vi "Draw Line - Octant 1.vi"(5 "Delta y":i32, 6 "Colour":u32(colorbox), 7 "Delta x":i32, 8 "x Direction":i32, 9 "Y0":i32, 10 "X0":i32, 11 "Pixel Data in":u32[][](array[numeric])) -> (3 "Pixel Data out":u32[][](array[numeric]))   [LabVIEW 2022 SP3, in "Raster.lvlib"]
uses:
  Raster.lvlib
  Utility/Convert Pixels To Picture.vi/d601d993-a776-4dc8-89c7-357d8398c88c.vi
  Utility/Convert Pixels To Picture.vi/7816d0d6-8e4d-41a2-85ac-ed82f1435763.vi
  <vilib>/Utility/High Resolution Relative Seconds.vi
  <vilib>/picture/picture.llb/Draw Unflattened Pixmap.vi
  <vilib>/picture/picture.llb/Draw True-Color Pixmap.vi
  Utility/Utility.lvlib
panel:
  out "new picture 2":picture
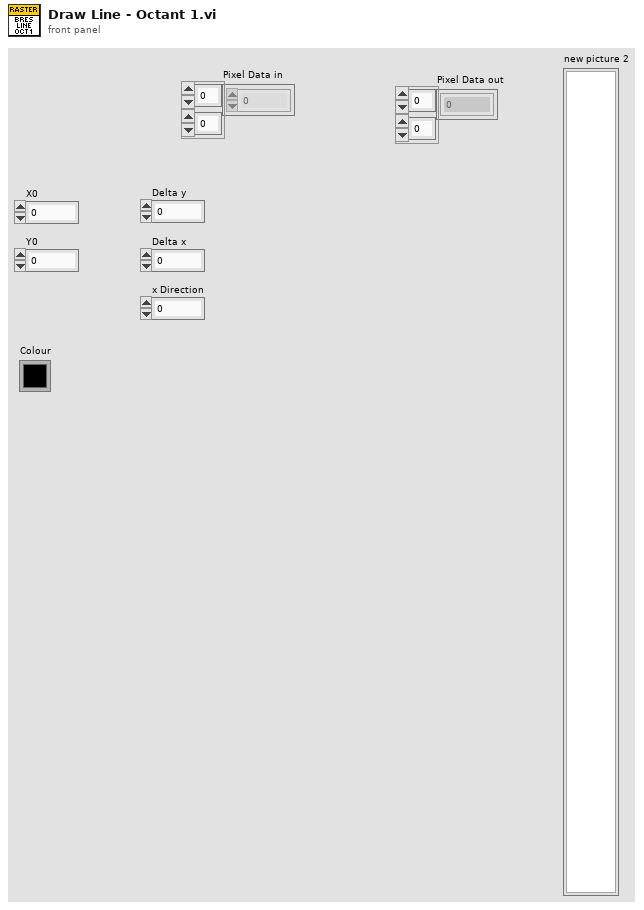
[diagram p1: front panel]
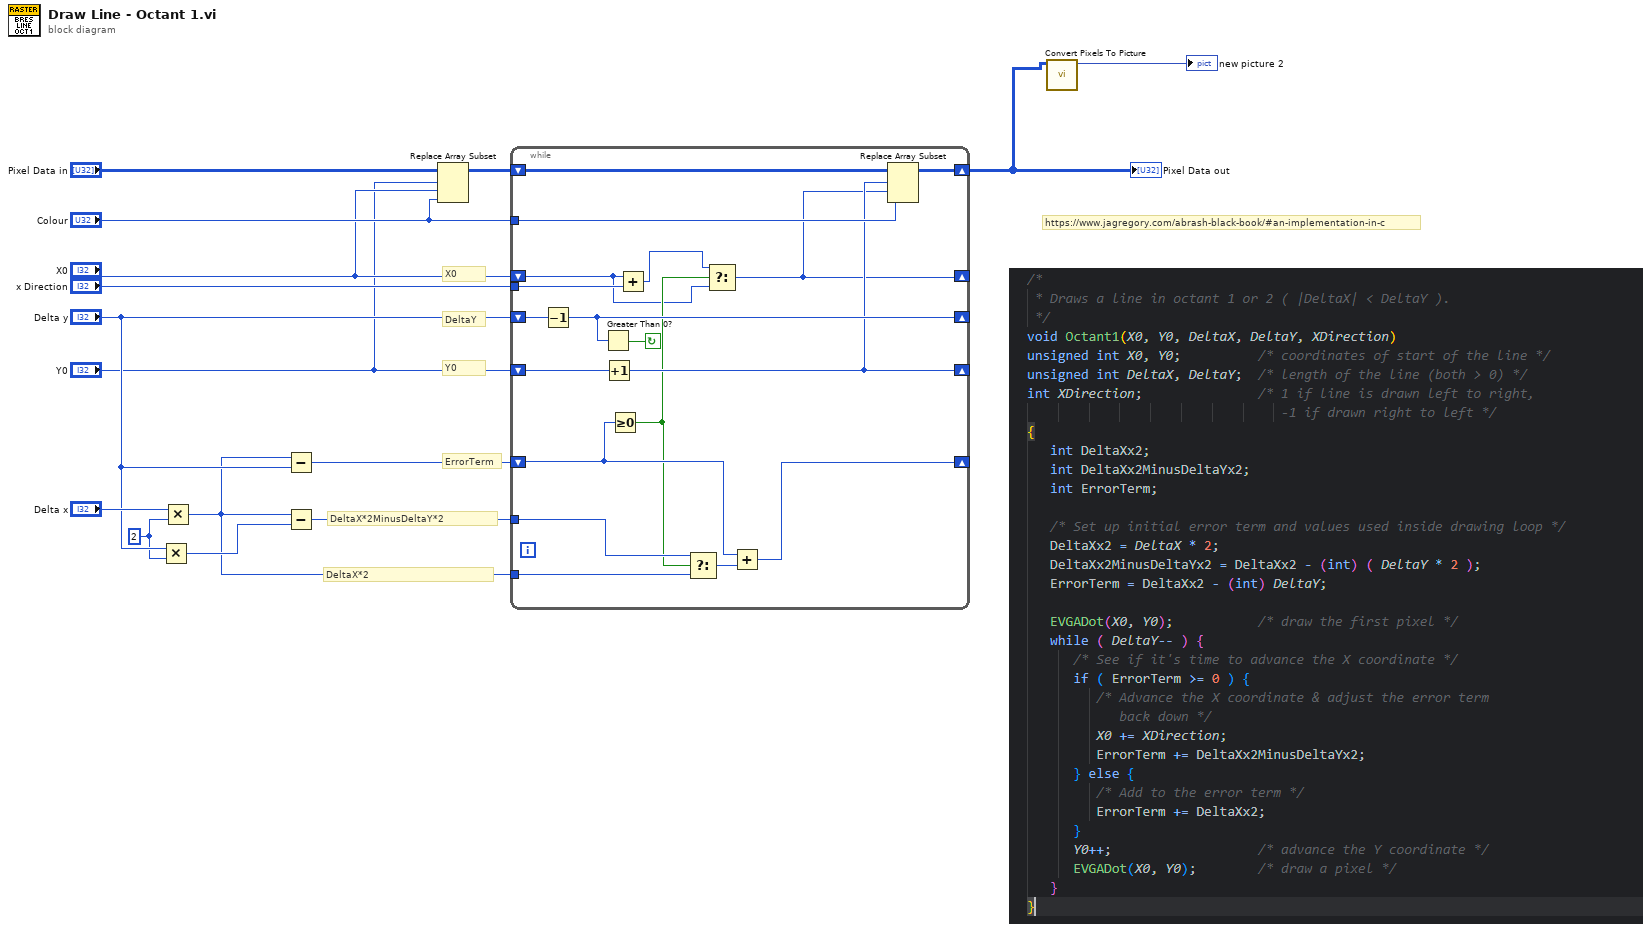
[diagram p0: block diagram]
diagram:
  w6 = 2 ("y")
  # "DeltaX*2"
  # "DeltaX*2MinusDeltaY*2"
  # "Y0"
  # "X0"
  # "DeltaY"
  # "https://www.jagregory.com/abrash-black-book/#an-implementation-in-c"
  # "ErrorTerm"
  n1 = Multiply(x="Delta y", y=w6) -> (x*y=w14:i32)
  n2 = Multiply(x="Delta x", y=w6) -> (x*y=w9:i32)
  n3 = Subtract(x=w9, y="Delta y") -> (x-y=w12:i32)
  n4 = Subtract(x=w9, y=w14) -> (x-y=w10:i32)
  n5 = Replace Array Subset(array="Pixel Data in", new element="Colour", index (row)="Y0", index (col)="X0") -> (w13:u32[][])
  n6 = while {
    shift-right: [w29] -> w1
    shift-left: w13 -> [w30]
    shift-right: [w31] -> _
    shift-left: w12 -> [w24]
    shift-right: [w26] -> _
    shift-left: "Delta y" -> [w33]
    shift-right: [w17] -> _
    shift-left: "X0" -> [w16]
    shift-right: [w20] -> _
    shift-left: "Y0" -> [w21]
    tunnel: w10 -> [w25]
    tunnel: w9 -> [w22]
    tunnel: "x Direction" -> [w28]
    tunnel: "Colour" -> [w27]
    stop <- w32 continue-if-true
    n7 = Decrement(x=w33) -> (x-1=w26:i32)
    n8 = Greater Than 0?(x=w26) -> (x > 0?=w32:bool)
    n9 = Increment(x=w21) -> (x+1=w20:i32)
    n10 = Greater Or Equal To 0?(x=w24) -> (x >= 0?=w19:bool)
    n11 = Add(x=w16, y=w28) -> (x+y=w18:i32)
    n12 = Select(t=w25, s=w19, f=w22) -> (s? t:f=w23:i32)
    n13 = Select(t=w18, s=w19, f=w16) -> (s? t:f=w17:i32)
    n14 = Add(x=w24, y=w23) -> (x+y=w31:i32)
    n15 = Replace Array Subset(array=w30, new element=w27, index (row)=w20, index (col)=w17) -> (w29:u32[][])
  }
  "Pixel Data out" <- w1
  n16 = call "Convert Pixels To Picture.vi"("Pixel Data in"=w1) -> ("2D Picture"=→"new picture 2":picture)  [unwired: 9 in, 1 out]
